vi "Configure Output Rate.vi"(8 "Error in (no error)":errorcluster, 10 "Output Rate ( 4 )":i32=4 min=-50 max=40 step=1, 11 "VISA resource name":refnum<visa-resource-name>) -> (0 "Error out":errorcluster, 3 "VISA resource out":refnum<visa-resource-name>)   [LabVIEW 2011, in "Ocean Server OS4000.lvlib"]
doc: "Set the compass output rate, -50 to +40"
uses:
  Ocean Server OS4000.lvlib
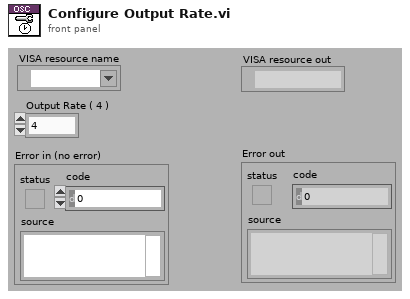
[diagram p1: front panel]
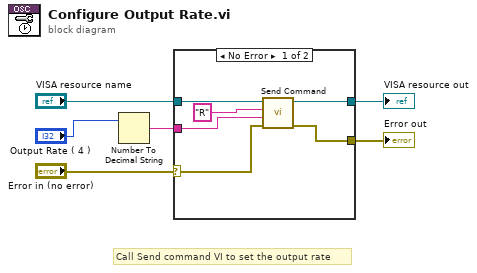
[diagram p0: block diagram]
diagram:
  # "Call Send command VI to set the output rate"
  n1 = Number To Decimal String(number="Output Rate ( 4 )") -> (decimal integer string=w1:string)  [unwired: 1 in]
  n2 = case shown="No Error" "Error in (no error)" {
    selector: "Error in (no error)" -> [w11 w14]
    tunnel: "VISA resource name" -> [w12 w13]
    tunnel: [w10 w14] -> w4
    tunnel: [w9 w13] -> w3
    tunnel: w1 -> [w7 _]
    frame No Error {
      n3 = call "Send Command.vi"("error in (no error)"=w11, "Value"=w7, "Message"="R", "VISA resource name"=w12) -> ("error out"=w10:errorcluster, "VISA resource out"=w9:refnum<visa-resource-name>)  [unwired: 6 in]
    }
    frame Error {
    }
  }
  "Error out" <- w4
  "VISA resource out" <- w3
